vi "searchROSMsg.vi"(3 "type":string) -> (0 "error out":errorcluster, 1 "File":string)   [LabVIEW 2015]
panel:
  out "folder names":string[](array[string])
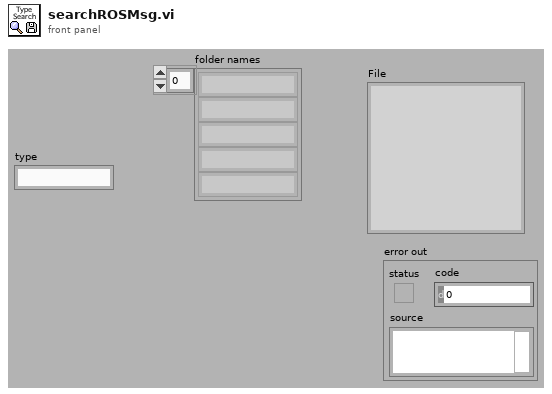
[diagram p1: front panel]
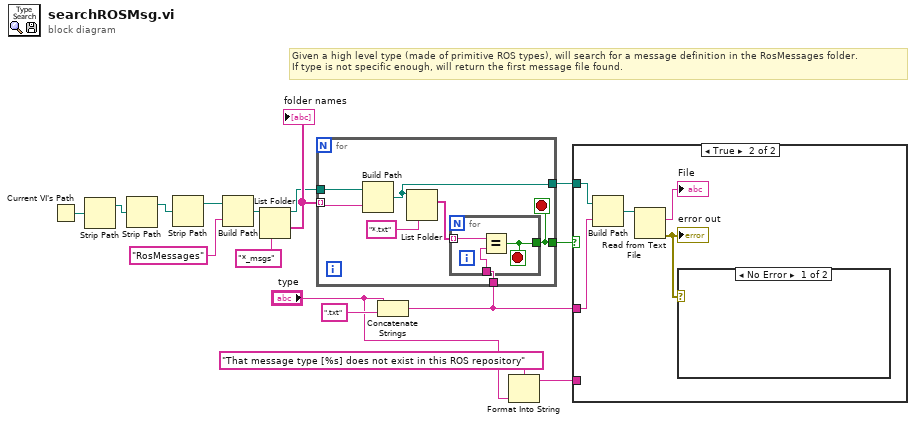
[diagram p0: block diagram]
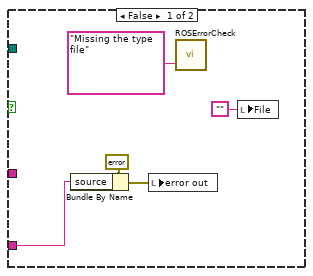
[diagram p2: hidden frame]
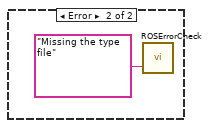
[diagram p3: hidden frame]
diagram:
  # "Given a high level type (made of primitive ROS types), will search for a message definition in the RosMessages folder.\nIf type is not specific enough, will return the first message file found."
  n1 = Current VI's Path() -> (path=w16:path)
  n2 = Strip Path(path=w16) -> (stripped path=w13:path)  [unwired: 1 out]
  n3 = Strip Path(path=w13) -> (stripped path=w12:path)  [unwired: 1 out]
  n4 = Strip Path(path=w12) -> (stripped path=w14:path)  [unwired: 1 out]
  n5 = Build Path(base path=w14, name or relative path="RosMessages" ("string")) -> (appended path=w11:path)
  n6 = List Folder(path=w11, pattern="*_msgs") -> (path out=w4:path, folder names=w5:string[])  [unwired: 2 in, 2 out]
  "folder names" <- w5
  n7 = Concatenate Strings("type", ".txt" ("string")) -> (w1:string)
  n8 = for {
    tunnel: w5 -> [w22] mode=indexing
    tunnel: w4 -> [w23]
    tunnel: w1 -> [w19]
    tunnel: [w18] -> w3
    tunnel: [w17] -> w2
    stop <- w18 stop-if-true
    n9 = Build Path(base path=w23, name or relative path=w22) -> (appended path=w17:path)
    n10 = List Folder(path=w17, pattern="*.txt") -> (filenames=w20:string[])  [unwired: 2 in, 3 out]
    n11 = for {
      tunnel: w20 -> [w26] mode=indexing
      tunnel: w19 -> [w25]
      tunnel: [w24] -> w18
      stop <- w24 stop-if-true
      n12 = Equal?(x=w26, y=w25) -> (x = y?=w24:bool)
    }
  }
  n13 = Format Into String(format string="That message type [%s] does not exist in this ROS repository" ("source"), "type") -> (resulting string=w8:string)  [unwired: 2 in, 1 out]
  n14 = case shown="True" w3 {
    tunnel: w8 -> [w27 _]
    tunnel: w2 -> [_ w33]
    tunnel: w1 -> [_ w32]
    frame False {
      n15 = Bundle By Name(cluster=errorcluster {"status"=TRUE, "code"=0, "source"=""} ("error out"), "source"=w27) -> (w28:errorcluster)
      n16 = local write "error out"(w28) -> ()
      n17 = call "ROSErrorCheck.vi"("message"="Missing the type file") -> ()  [unwired: 2 in, 1 out]
      n18 = local write "File"("" ("File")) -> ()
    }
    frame True {
      n19 = Build Path(base path=w33, name or relative path=w32) -> (appended path=w36:path)
      n20 = Read from Text File(file (use dialog)=w36) -> (text=→"File":string, error out=w34:errorcluster)  [unwired: 3 in, 2 out]
      "error out" <- w34
      n21 = case shown="No Error" w34 {
        frame No Error {
        }
        frame Error {
          n22 = call "ROSErrorCheck.vi"("message"="Missing the type file") -> ()  [unwired: 2 in, 1 out]
        }
      }
    }
  }
